vi "SortByID.vi"(5 "Headers":string[](array[string])=["Timestamp", "ID", "Type", "Dir", "DLC", "Data"], 7 "Trace":refnum<vi>, 8 "error in":errorcluster, 9 "Unsorted Data":string[][](array[string]), 10 "SortByID":refnum<vi>, 11 "Filter":refnum<vi>) -> (0 "error out":errorcluster, 3 "Table Control":string[][](array[string]))   [LabVIEW 2025, in "CAN-LIN Raw Bus Capture UI.lvlib"]
doc: "Filters and Shorts the Table, and updates it's values with the sorted filtered data."
uses:
  CAN-LIN Raw Bus Capture UI.lvlib
  Table_Filtering/Table_Filtering.lvlib
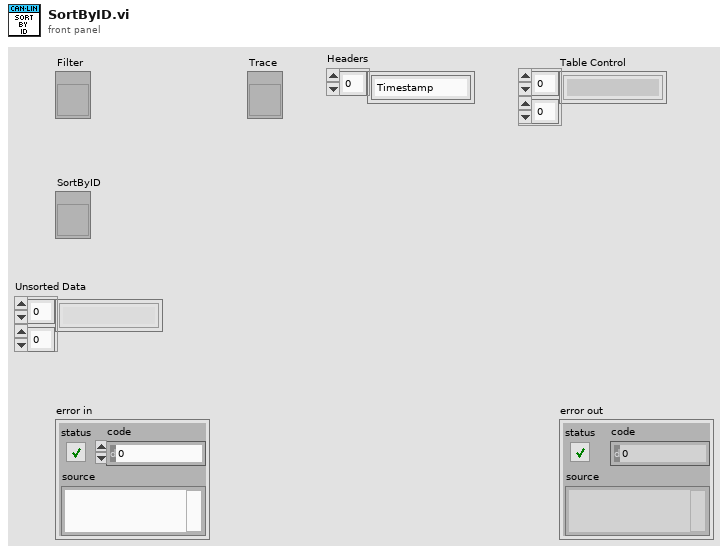
[diagram p1: front panel]
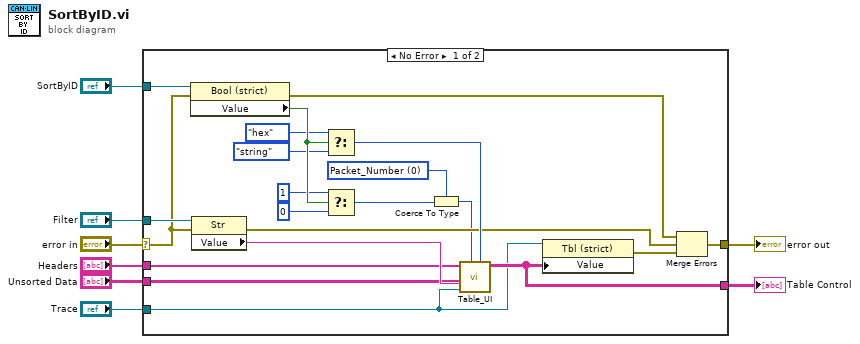
[diagram p0: block diagram]
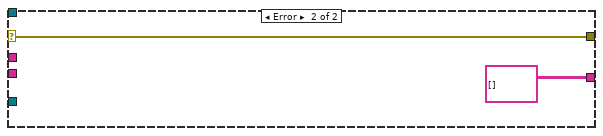
[diagram p2: hidden frame]
diagram:
  n1 = case shown="No Error" "error in" {
    selector: "error in" -> [w19 w31]
    tunnel: [w18 string[][] [] ("Table Control")] -> w8
    tunnel: [w22 w31] -> w6
    tunnel: "Filter" -> [w21 _]
    tunnel: "SortByID" -> [w20 _]
    tunnel: "Trace" -> [w10 _]
    tunnel: "Headers" -> [w17 _]
    tunnel: "Unsorted Data" -> [w9 _]
    frame No Error {
      w13 = u16 0 items=["Packet_Number", "Timestamp", "Source", "Destination", "Protocol", "Length", "Data"] ("Sort by")
      n2 = property class="Bool (strict)"(reference=w20, error in=w19) -> (error out=w16:errorcluster, "Value"=w29:bool)  [unwired: 1 out]
      n3 = property class="Str"(reference=w21, error in=w19) -> (error out=w15:errorcluster, "Value"=w28:string)  [unwired: 1 out]
      n4 = Select(t=enum16{"numerical", "hex", "string"}."hex" ("Sort Type"), s=w29, f=enum16{"numerical", "hex", "string"}."string" ("Sort Type")) -> (s? t:f=w23:enum16{"numerical", "hex", "string"})
      n5 = Select(t=1, s=w29, f=0) -> (s? t:f=w12:i32)
      n6 = Coerce To Type(0:w12, 1:w13) -> (2:w11:u16)
      n7 = call "Table_UI.vi"("Sort Type"=w23, "Sort by"=w11, "Table Control"=w10, "Unsorted Data"=w9, "Filter String"=w28, "Headers"=w17) -> ("Table Control"=w18:string[][])  [unwired: 5 in]
      n8 = property on="Property Node" class="Tbl (strict)"(reference=w10, "Value"=w18) -> (error out=w14:errorcluster)  [unwired: 1 in, 1 out]
      n9 = Merge Errors(w16, w15, w14) -> (w22:errorcluster)
    }
    frame Error {
    }
  }
  "error out" <- w6
  "Table Control" <- w8
